vi "dfd_Convert String to Complex Array .vi"(8 "error in":errorcluster, 11 "string":string) -> (0 "error out":errorcluster, 3 "roots":cdb[](array[numeric]))   [LabVIEW 2017, in "NI_DigFilter_Process.lvlib"]
uses:
  <vilib>/addons/Digital Filter Design/NI_DigFilter_Process.lvlib
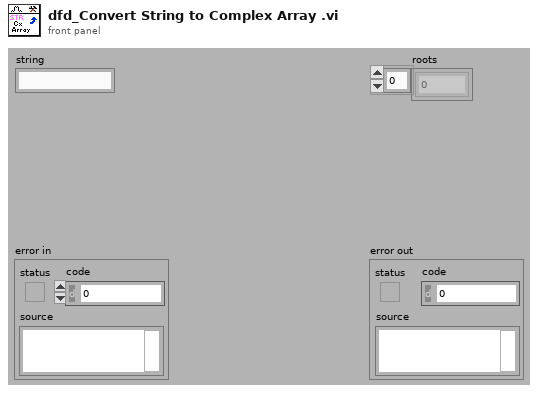
[diagram p1: front panel]
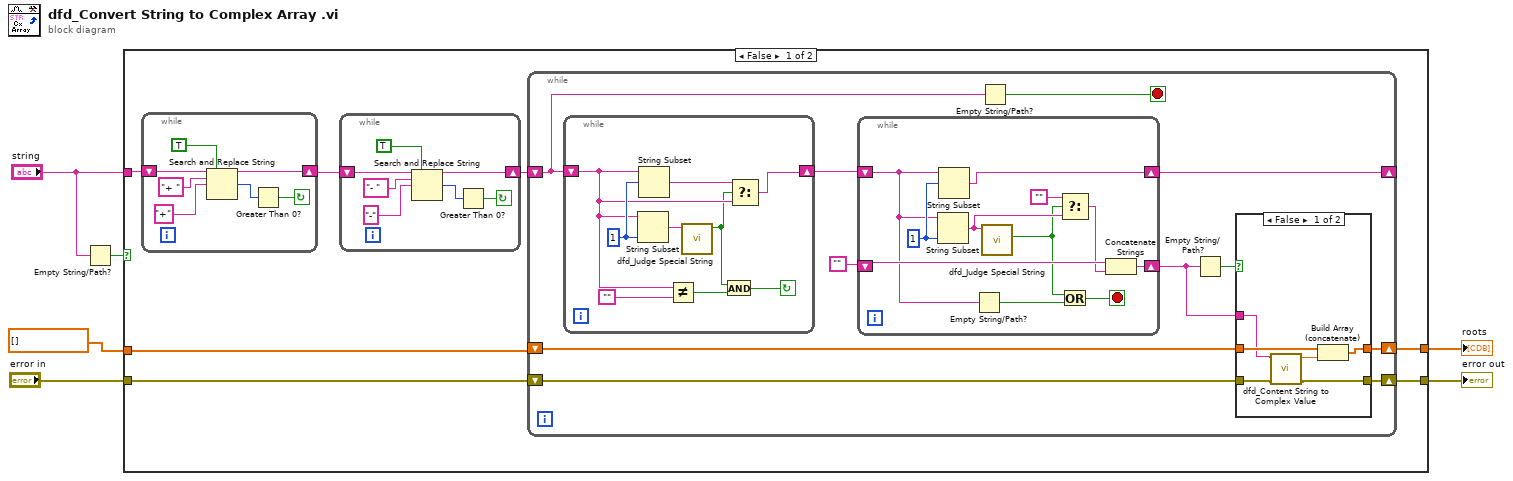
[diagram p0: block diagram]
diagram:
  n1 = Empty String/Path?(string/path="string") -> (empty?=w3:bool)
  n2 = case shown="False" w3 {
    tunnel: "string" -> [w8 _]
    tunnel: [w13 w68] -> w6
    tunnel: "error in" -> [w12 w67]
    tunnel: [w11 w67] -> w4
    tunnel: cdb[] [] ("roots") -> [w10 w68]
    frame False {
      n3 = while {
        shift-right: [w27] -> w9
        shift-left: w8 -> [w26]
        stop <- w24 continue-if-true
        n4 = Search and Replace String(replace all?=TRUE ("replace all? (F)"), input string=w26, search string="+ ", replace string="+") -> (result string=w27:string, number of replacements=w25:i32)  [unwired: 1 in, 5 out]
        n5 = Greater Than 0?(x=w25) -> (x > 0?=w24:bool)
      }
      n6 = while {
        shift-right: [w20] -> w7
        shift-left: w9 -> [w19]
        stop <- w17 continue-if-true
        n7 = Search and Replace String(replace all?=TRUE ("replace all? (F)"), input string=w19, search string="- ", replace string="-") -> (result string=w20:string, number of replacements=w18:i32)  [unwired: 1 in, 5 out]
        n8 = Greater Than 0?(x=w18) -> (x > 0?=w17:bool)
      }
      n9 = while {
        shift-right: [w38] -> _
        shift-left: w7 -> [w35]
        shift-right: [w31] -> w11
        shift-left: w12 -> [w30]
        shift-right: [w29] -> w13
        shift-left: w10 -> [w28]
        stop <- w34 stop-if-true
        n10 = while {
          shift-right: [w64] -> w37
          shift-left: w35 -> [w62]
          stop <- w59 continue-if-true
          w66 = 1 ("length (rest)")
          n11 = String Subset(string=w62, length (rest)=w66) -> (substring=w63:string)  [unwired: 1 out]
          n12 = String Subset(string=w62, offset (0)=w66) -> (substring=w65:string)  [unwired: 1 out]
          n13 = Not Equal?(x=w62, y="") -> (x != y?=w61:bool)
          n14 = call <vilib>:"dfd_Judge Special String.vi"("string"=w63) -> ("space ?"=w60:bool)  [unwired: 10 out]
          n15 = And(x=w60, y=w61) -> (x .and. y?=w59:bool)
          n16 = Select(t=w65, s=w60, f=w62) -> (s? t:f=w64:string)
        }
        n17 = while {
          shift-right: [w55] -> w38
          shift-left: w37 -> [w50]
          shift-right: [w51] -> w32
          shift-left: "" -> [w56]
          stop <- w47 stop-if-true
          w57 = 1 ("length (rest)")
          n18 = String Subset(string=w50, length (rest)=w57) -> (substring=w54:string)  [unwired: 1 out]
          n19 = String Subset(string=w50, offset (0)=w57) -> (substring=w55:string)  [unwired: 1 out]
          n20 = Empty String/Path?(string/path=w50) -> (empty?=w49:bool)
          n21 = call <vilib>:"dfd_Judge Special String.vi"("string"=w54) -> ("separator"=w48:bool)  [unwired: 10 out]
          n22 = Select(t="", s=w48, f=w54) -> (s? t:f=w53:string)
          n23 = Or(x=w48, y=w49) -> (x .or. y?=w47:bool)
          n24 = Concatenate Strings(w56, w53) -> (w51:string)
        }
        n25 = Empty String/Path?(string/path=w35) -> (empty?=w34:bool)
        n26 = Empty String/Path?(string/path=w32) -> (empty?=w33:bool)
        n27 = case shown="False" w33 {
          tunnel: w32 -> [w41 _]
          tunnel: [w39 w45] -> w31
          tunnel: w30 -> [w40 w45]
          tunnel: [w44 w46] -> w29
          tunnel: w28 -> [w43 w46]
          frame False {
            n28 = call <vilib>:"dfd_Content String to Complex Value.vi"("error in (no error)"=w40, "string"=w41) -> ("error out"=w39:errorcluster, "value"=w42:cdb)  [unwired: 8 out]
            n29 = Build Array (concatenate)(w43, w42) -> (w44:cdb[])
          }
          frame True {
          }
        }
      }
    }
    frame True {
    }
  }
  "roots" <- w6
  "error out" <- w4
